vi "Car Wash.vi"() -> ()   [LabVIEW 2015]
uses:
  Controls/Car Wash Indicators.ctl
  Controls/Wash Options.ctl
  MHL Data.ctl
  User Interface Data.ctl
  SupportVIs/Queues/Message.ctl
  <vilib>/Utility/file.llb/Read Delimited Spreadsheet (I64).vi
panel:
  in  "Start":bool
  out "Elapsed Time":dbl format="%0.2f"
  in  "stop":bool
  out "Wash Entry":bool
  in  "Wash Options":T1
  out "Car Position Slider":u8(slide) max=3 scale=0.0..4.0
  out "Car Wash Indicators":T2
  # "Entry Console"
  # "Car Wash Display"
  # "Car Position Simulation"
  # "Pre-Soak\nH-P Wash\nL-P Wax\nSpot Free Rinse"
  # "Underbody Wash\nBug Remover"
  # "Tire Shine\nAir Dry"
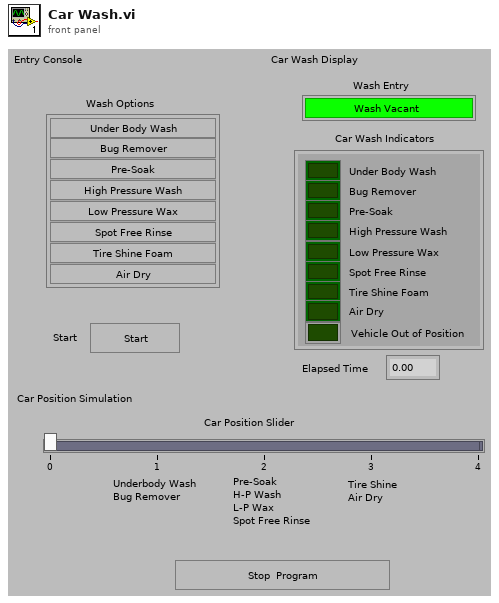
[diagram p1: front panel]
types:
  T1 = typedef "Wash Options.ctl" = cluster{"Underbody Wash":bool, "Bug Remover":bool, "Pre-Soak":bool, "High Pressure Wash":bool, "Low Pressure Wax":bool, "Spot Free Rinse":bool, "Tire Shine Foam":bool, "Air Dry":bool}
  T2 = typedef "Car Wash Indicators.ctl" = cluster{"Under Body Wash":bool, "Bug Remover":bool, "Pre-Soak":bool, "High Pressure Wash":bool, "Low Pressure Wax":bool, "Spot Free Rinse":bool, "Tire Shine Foam":bool, "Air Dry":bool, "Vehicle Out of Position":bool}
  T3 = typedef "MHL Data.ctl" = cluster{"User Iterface Data":T4, "MHL References":cluster{"Wash Options":refnum<vi>, "Start":refnum<vi>, "stop":refnum<vi>}}
  T4 = typedef "User Interface Data.ctl" = cluster{"Car Position Slider":u8, "Car Wash Indicators":T2, "Elapsed Time":dbl, "Wash Entry":bool}
  T5 = typedef "Message Queues.ctl" = cluster{"MHL Queue":refnum<queue>, "Washing Queue ":refnum<queue>}
  T6 = typedef "Message.ctl" = enum16{"UpdateDisplay", "Run Washing", "Exit", "Initialize"}
  T7 = cluster{"Wash Options":refnum<vi>, "Start":refnum<vi>, "stop":refnum<vi>}
  T8 = cluster{"Car Position Slider":u8, "Car Wash Indicators":T2, "Elapsed Time":dbl, "Wash Entry":bool}
  T9 = typedef "Washing Control Cluster.ctl" = cluster{"Message Data":variant, "States of Washing":T10}
  T10 = typedef "States of Washing.ctl" = enum16{"Start", "Under Body Wash", "Bug Remover", "Pre-Soak", "High Pressure Wax", "Low Pressure Wax", "Spot Free Rinse", "Tire Shine Foam", "Air Dry", "End", "Initialize"}
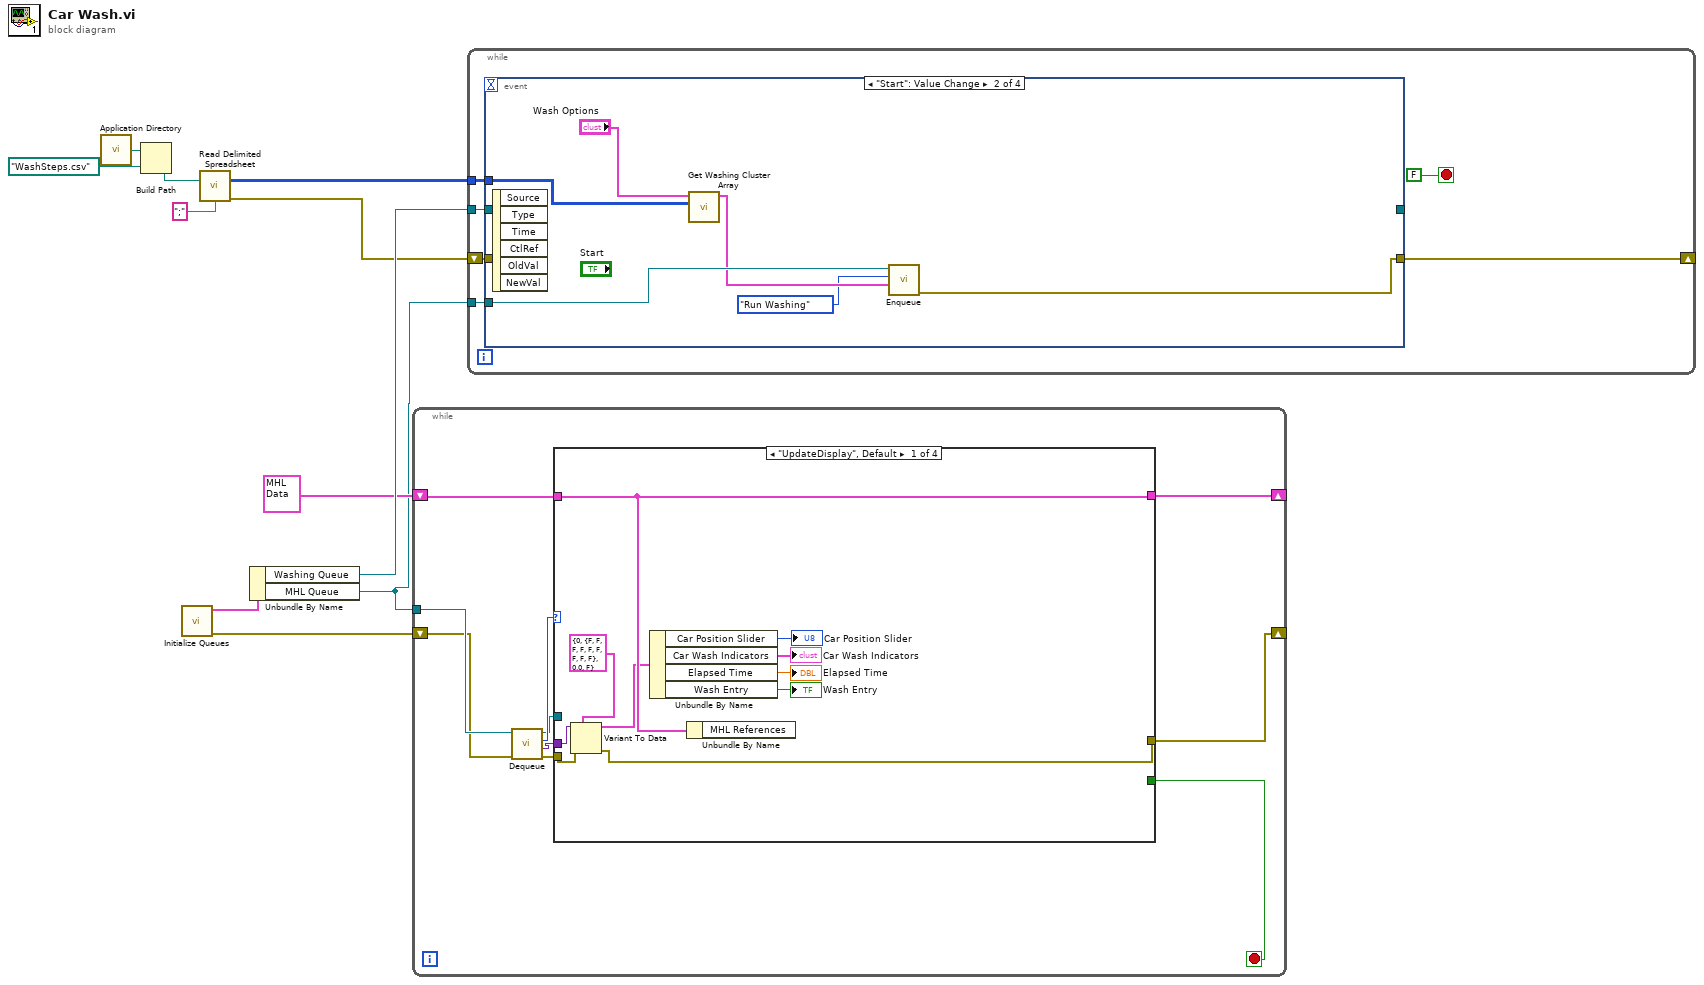
[diagram p0: block diagram]
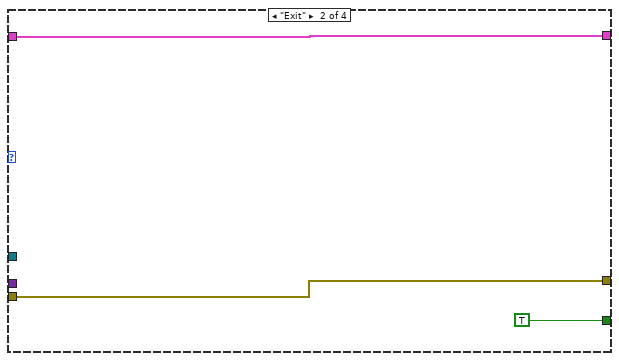
[diagram p2: hidden frame]
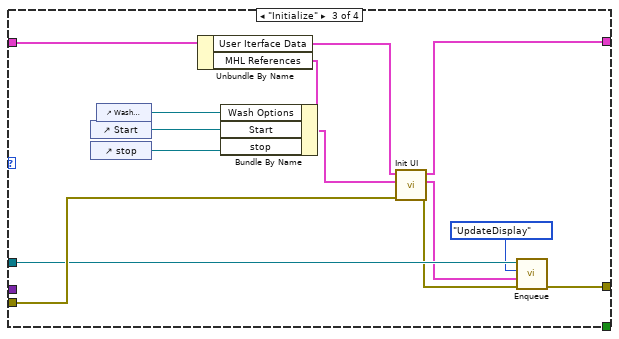
[diagram p3: hidden frame]
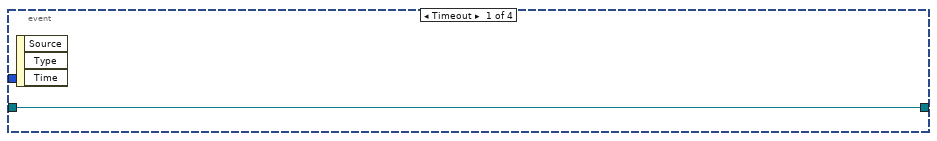
[diagram p5: hidden frame]
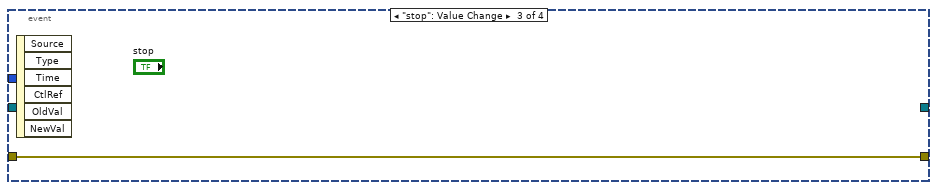
[diagram p6: hidden frame]
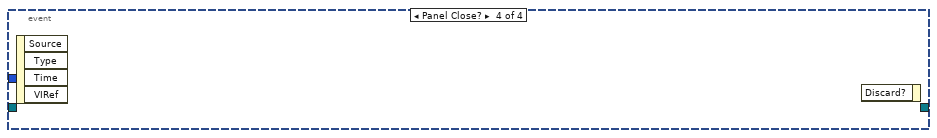
[diagram p7: hidden frame]
diagram:
  n1 = call <vilib>:"Application Directory.vi"() -> ("Application Directory"=w2:path)
  n2 = Build Path(base path=w2, name or relative path=path "WashSteps.csv" ("file path (use dialog)")) -> (appended path=w6:path)
  n3 = call "Initialize Queues.vi"() -> ("error out"=w9:errorcluster, "output cluster"=w11:T5)  [unwired: 10 in]
  n4 = call-poly <vilib>:"Read Delimited Spreadsheet.vi"("file path (dialog if empty)"=w6, "delimiter (\\t)"=";" ("delimiter (\\t)")) -> ("all rows"=w4:i64[][], "error out"=w1:errorcluster)  [unwired: 8 in, 4 out]
  n5 = Unbundle By Name(w11) -> ("Washing Queue"=w10:refnum<queue>, "MHL Queue"=w3:refnum<queue>)
  n6 = while {
    tunnel: w3 -> [w21]
    shift-right: [w18] -> _
    shift-left: w9 -> [w17]
    shift-right: [w15] -> _
    shift-left: T3 {"User Iterface Data"={"Car Position Slider"=0, "Car Wash Indicators"={"Under Body Wash"=FALSE, "Bug Remover"=FALSE, "Pre-Soak"=FALSE, "High Pressure Wash"=FALSE, "Low Pressure Wax"=FALSE, "Spot Free Rinse"=FALSE, "Tire Shine Foam"=FALSE, "Air Dry"=FALSE, "Vehicle Out of Position"=FALSE}, "Elapsed Time"=0.0, "Wash Entry"=FALSE}, "MHL References"={"Wash Options"=refnum, "Start"=refnum, "stop"=refnum}} ("MHL Data") -> [w14]
    stop <- w19 stop-if-true
    n7 = call "Dequeue.vi"("error in (no error)"=w17, "Message Queue in"=w21) -> ("error out"=w16:errorcluster, "Message Data"=w12:variant, "Message"=w20:T6, "Message Queue out"=w13:refnum<queue>)  [unwired: 6 in]
    n8 = case shown="\"UpdateDisplay\", Default" w20 {
      tunnel: [_ TRUE _ _] -> w19
      tunnel: w16 -> [w23 w33 w48 w50]
      tunnel: [w22 w33 w35 w50] -> w18
      tunnel: [w30 w32 w40 w49] -> w15
      tunnel: w14 -> [w30 w32 w47 w49]
      tunnel: w13 -> [_ _ w39 _]
      tunnel: w12 -> [w31 _ _ _]
      frame "UpdateDisplay", Default {
        n9 = Variant To Data(error in=w23, type=T4 {"Car Position Slider"=0, "Car Wash Indicators"={"Under Body Wash"=FALSE, "Bug Remover"=FALSE, "Pre-Soak"=FALSE, "High Pressure Wash"=FALSE, "Low Pressure Wax"=FALSE, "Spot Free Rinse"=FALSE, "Tire Shine Foam"=FALSE, "Air Dry"=FALSE, "Vehicle Out of Position"=FALSE}, "Elapsed Time"=0.0, "Wash Entry"=FALSE} ("User Iterface Data"), Variant=w31) -> (data=w28:T4, error out=w22:errorcluster)
        n10 = Unbundle By Name(w28) -> ("Car Position Slider"=→"Car Position Slider":u8, "Car Wash Indicators"=→"Car Wash Indicators":T2, "Elapsed Time"=→"Elapsed Time":dbl, "Wash Entry"=→"Wash Entry":bool)
        n11 = Unbundle By Name(w30) -> ()  [unwired: 1 out]
      }
      frame "Exit" {
      }
      frame "Initialize" {
        n12 = control-ref of="Start"() -> (w44:refnum<vi>)
        n13 = control-ref of="stop"() -> (w43:refnum<vi>)
        n14 = control-ref of="Wash Options"() -> (w45:refnum<vi>)
        n15 = Unbundle By Name(w47) -> ("User Iterface Data"=w42:T4, "MHL References"=w46:T7)
        n16 = Bundle By Name(cluster=w46, "Wash Options"=w45, "Start"=w44, "stop"=w43) -> (w41:T7)
        n17 = call "Init UI.vi"("error in (no error)"=w48, "MHL References"=w41, "User Iterface Data"=w42) -> ("error out"=w36:errorcluster, "User Iterface Data out"=w38:T8, "MHL Data"=w40:T3)  [unwired: 4 in]
        n18 = call "Enqueue.vi"("error in (no error)"=w36, "Message Data"=w38, "Message"=Message."UpdateDisplay", "Message Queue"=w39) -> ("error out"=w35:errorcluster)  [unwired: 6 in, 1 out]
      }
      frame "Run Washing" {
      }
    }
  }
  n19 = while {
    tunnel: w10 -> [w56]
    shift-right: [w53] -> _
    shift-left: w1 -> [w54]
    tunnel: w4 -> [w52]
    tunnel: w3 -> [w51]
    stop <- FALSE stop-if-true
    n20 = event shown="[1] \"Start\": Value Change" {
      selector: _ -> [_ _ _ _]
      dyn-events: _ -> [_ _ _ _]
      timeout: _ -> [_ _ _ _]
      tunnel: [w57 _ _ _] -> _
      tunnel: w56 -> [w57 _ _ _]
      tunnel: [_ w58 w64 _] -> w53
      tunnel: w54 -> [_ _ w64 _]
      tunnel: w52 -> [_ w62 _ _]
      tunnel: w51 -> [_ w61 _ _]
      event Timeout {
        n21 = event-data() -> ()  [unwired: 1 in, 3 out]
      }
      event "Start": Value Change {
        n22 = event-data() -> ()  [unwired: 1 in, 6 out]
        n23 = call "Get Washing Cluster Array.vi"("all rows"=w62, "Wash Options"="Wash Options") -> ("Array"=w60:T9[])  [unwired: 9 in]
        n24 = call "Enqueue.vi"("Message Data"=w60, "Message"=Message."Run Washing", "Message Queue"=w61) -> ("error out"=w58:errorcluster)  [unwired: 7 in, 1 out]
      }
      event "stop": Value Change {
        n25 = event-data() -> ()  [unwired: 1 in, 6 out]
      }
      event Panel Close? {
        n26 = event-data() -> ()  [unwired: 1 in, 4 out]
        n27 = event-data() -> ()  [unwired: 2 in, 1 out]
      }
    }
  }
